vi "GLIMPSE Save image.vi"(5 "Go? (F)":bool, 7 "Header data":T1 {"Pixel depth" items=["8 bits", "16 bits", "Float", "Complex", "RGB", "HSL"]; "time of 1st frame, \nsec since 1/1/04" format="%.2f"}, 8 "Comment (for IMG file)":string, 9 "Acqisition files refnums":refnum<file>[](array[refnum]), 10 "Frame number":u32) -> (3 "Saved Image":T5)   [LabVIEW 2011]
uses:
  <vilib>/vision/Image Controls.llb/IMAQ Image.ctl
  Header file data.ctl
  Seq file v 1/Offset table.ctl
  Seq file v 1/Offset.ctl
  Seq file v 1/file number.ctl
  GLIMPSE Globals.vi
  <vilib>/vision/NI_Vision_Development_Module.lvlib
panel:
  out "Global Rectangle":i32[](array[numeric])
  in  "file path":path
  in  "File format":enum16{"TIFF", "IMG"}(ring)
  in  "stop":bool
  # "Designate an AOI to save, then press GO.\nIf no AOI is selected, the whole image will be saved."
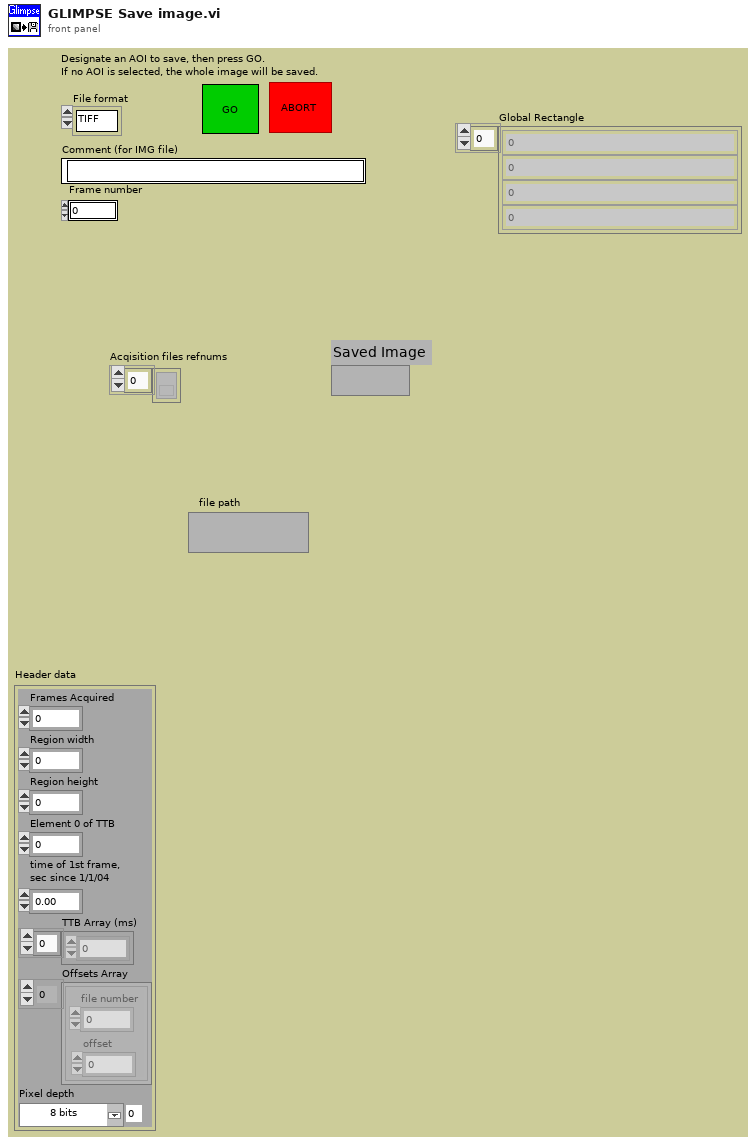
[diagram p1: front panel]
types:
  T1 = typedef "Header file data.ctl" = cluster{"Frames Acquired":u32, "Region width":i32, "Region height":i32, "Element 0 of TTB":u32, "time of 1st frame, \nsec since 1/1/04":dbl, "TTB Array (ms)":u32[], "Offsets Array":T2, "Pixel depth":u32}
  T2 = typedef "Offset table.ctl" = cluster{"offset":T3, "file number":T4}[]
  T3 = typedef "Offset.ctl" = i32
  T4 = typedef "file number.ctl" = u8
  T5 = typedef "IMAQ Image.ctl" = refnum<image>
  T6 = enum32{"No Selection", "Point", "Line", "Rectangle", "Oval", "Polygon", "Free", "Unused1", "Zoom", "Unused2", "Broken Line", "Free Hand Line"}
  T7 = enum16{"open", "open or create", "create or replace", "create"}
  T8 = enum32{"No Selection", "Point", "Line", "Rectangle", "Oval", "Polygon", "Free", "Unused1", "Zoom", "Unused2", "Broken Line", "Free Hand Line"}[]
  T9 = typedef "ROI Descriptor" = cluster{"Global Rectangle":i32[], "Contours":cluster{"ID":enum32{"External", "Internal"}, "Type":u32, "Coordinates":i32[]}[]}
  T10 = cluster{i32, i32, "X Resolution":i32, "Y Resolution":i32, dbl}
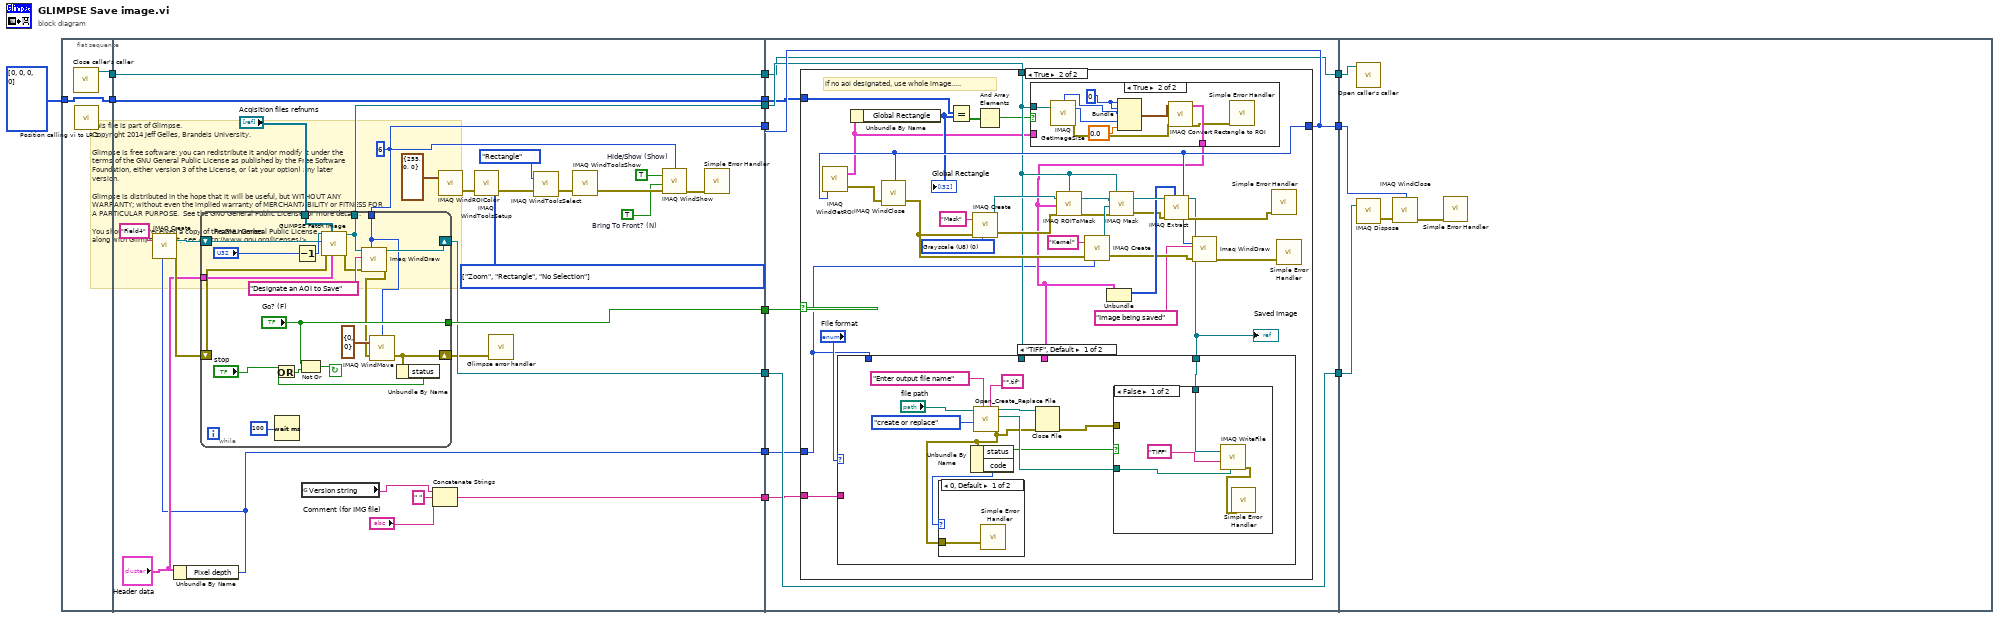
[diagram p0: block diagram]
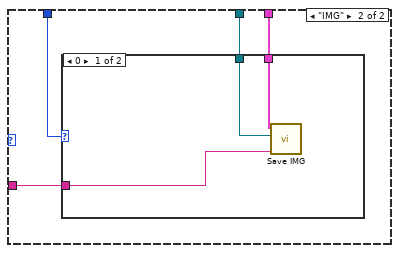
[diagram p6: hidden frame]
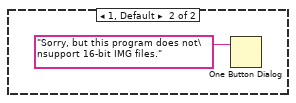
[diagram p7: hidden frame]
diagram:
  # "This file is part of Glimpse. \nCopyright 2014 Jeff Gelles, Brandeis University.    \n\nGlimpse is free software: you can redistribute it and/or modify it under the \nterms of the GNU General Public License as published by the Free Software \nFoundation, either version 3 of the License, or (at your option) any later \nversion.\n\nGlimpse is distributed in the hope that it will be useful, but WITHOUT ANY \nWARRANTY; without even the implied warranty of MERCHANTABILITY or FITNESS FOR \nA PARTICULAR PURPOSE.  See the GNU General Public License for more details.\n\nYou should have received a copy of the GNU General Public License\nalong with Glimpse.  If not, see <http://www.gnu.org/licenses/>."
  n1 = flat-sequence {
    tunnel: i32[] [0, 0, 0, 0] -> [w15]
    tunnel: [w15] -> w13
    tunnel: [w16] -> w12
    tunnel: w13 -> [w24]
    tunnel: [w24] -> w11
    tunnel: [w33] -> w10
    tunnel: [w31] -> w9
    tunnel: [w32] -> w8
    tunnel: [w28] -> w7
    tunnel: w12 -> [w23]
    tunnel: [w23] -> w6
    tunnel: [w19] -> w2
    tunnel: [w17] -> w1
    tunnel: w11 -> [w68]
    tunnel: w10 -> [w70]
    tunnel: w9 -> [w69]
    tunnel: w8 -> [w71]
    tunnel: [w71] -> w5
    tunnel: w7 -> [w67]
    tunnel: [w67] -> w4
    tunnel: w6 -> [w66]
    tunnel: [w66] -> w3
    tunnel: w2 -> [w65]
    tunnel: w1 -> [w64]
    tunnel: w5 -> [w138]
    tunnel: w4 -> [w136]
    tunnel: w3 -> [w135]
    frame #0 {
      n2 = call "Close caller's caller.vi"() -> ("vi reference"=w16:refnum<vi>)  [unwired: 1 in, 7 out]
      n3 = call "Position calling vi to LR 2.vi"() -> ()  [unwired: 2 in, 4 out]
    }
    frame #1 {
      w32 = 6 ("Window Number (0...15)")
      w35 = TRUE  # Bring To Front? (N)
      w36 = TRUE  # Hide/Show (Show)
      w41 = T8 [enum."Zoom", enum."Rectangle", enum."No Selection"] items=["No Selection", "Point", "Line", "Rectangle", "Oval", "Polygon", "Free", "Unused1", "Zoom", "Unused2", "Broken Line", "Free Hand Line"] ("Tools")
      n4 = Unbundle By Name("Header data") -> ("Pixel depth"=w17:u32)
      n5 = call "IMAQ Create"("Image Name"="Field4", "Image Type"=w17) -> ("New Image"=w29:T5, "error out"=w25:errorcluster)  [unwired: 2 in, 1 out]
      n6 = while {
        shift-left: w29 -> [w57]
        shift-right: [w55] -> w28
        tunnel: ["Go? (F)"] -> w31
        tunnel: w32 -> [w50]
        tunnel: [w58] -> w33
        tunnel: "Acqisition files refnums" -> [w53]
        shift-right: [w45] -> w26
        shift-left: w25 -> [w46]
        tunnel: "Header data" -> [w44]
        stop <- w62 continue-if-true
        n7 = Wait (ms)(milliseconds to wait=u32 100) -> ()  [unwired: 1 out]
        n8 = Decrement(x="Frame number") -> (x-1=w61:u32)
        n9 = call "GLIMPSE Fetch Image.vi"("Header file data"=w44, "Acqisition files refnums"=w53, "error in"=w46, "Logical Frame Number\n(starting with zero)"=w61, "Image In"=w57) -> ("error out"=w54:errorcluster, "Image Out"=w58:T5)  [unwired: 2 in, 3 out]
        n10 = call "Imaq WindDraw"("Window Number (0...15)"=w50, "error in (no error)"=w54, "Title"="Designate an AOI to Save", "Image"=w58) -> ("error out"=w51:errorcluster, "Image Out (duplicate)"=w55:T5)  [unwired: 2 in, 4 out]
        n11 = call "IMAQ WindMove"("Window Number (0...15)"=w50, "Coordinates (screen)"=cluster{"X Position":i32, "Y Position":i32} {"X Position"=0, "Y Position"=0}, "error in (no error)"=w51) -> ("error out"=w45:errorcluster)  [unwired: 1 in, 2 out]
        n12 = Unbundle By Name(w45) -> ("status"=w47:bool)
        n13 = Or(x="stop", y=w47) -> (x .or. y?=w49:bool)
        n14 = Not Or(1:w49, 2:"Go? (F)") -> (0:w62:bool)
      }
      n15 = global read "GLIMPSE Globals.vi" "Version string"() -> (w21:string)
      n16 = Concatenate Strings(w21, " " ("string"), "Comment (for IMG file)") -> (w19:string)
      n17 = call "IMAQ WindROIColor"("Color of ROI (white)"=cluster{"Red":u8, "Green":u8, "Blue":u8} {"Red"=255, "Green"=0, "Blue"=0}) -> ("error out"=w42:errorcluster)  [unwired: 1 in, 4 out]
      n18 = call "IMAQ WindToolsSetup"("Tools"=w41, "error in (no error)"=w42) -> ("error out"=w40:errorcluster)  [unwired: 2 in, 2 out]
      n19 = call "Glimpse error handler.vi"("error in"=w26) -> ()  [unwired: 1 in, 6 out]
      n20 = call "IMAQ WindToolsSelect"("Tool (Point)"=T6."Rectangle", "error in (no error)"=w40) -> ("error out"=w39:errorcluster)  [unwired: 2 in, 2 out]
      n21 = call "IMAQ WindToolsShow"("error in (no error)"=w39) -> ("error out"=w38:errorcluster)  [unwired: 2 in, 3 out]
      n22 = call "IMAQ WindShow"("error in (no error)"=w38, "Bring To Front? (N)"=w35, "Hide/Show (Show)"=w36, "Window Number (0...15)"=w32) -> ("error out"=w37:errorcluster)  [unwired: 1 in, 3 out]
      n23 = call <vilib>:"Simple Error Handler.vi"("error in (no error)"=w37) -> ()  [unwired: 1 in, 8 out]
    }
    frame #2 {
      n24 = case shown="True" w69 {
        tunnel: w71 -> [_ w87]
        tunnel: w70 -> [_ w79]
        tunnel: w68 -> [_ w76]
        tunnel: w65 -> [_ w74]
        tunnel: w64 -> [_ w73]
        frame False {
        }
        frame True {
          w72 = u32 0 items=["Grayscale (U8)", "Grayscale (I16)", "Grayscale (SGL)", "Complex (CSG)", "RGB (U32)", "HSL (U32)", "RGB (U64)"] ("Image Type")
          # "if no aoi designated, use whole image....."
          n25 = call "IMAQ WindGetROI"("Window Number (0...15)"=w87) -> ("ROI Descriptor"=w77:T9, "error out"=w100:errorcluster)  [unwired: 1 in, 3 out]
          n26 = Unbundle By Name(w77) -> ("Global Rectangle"=w81:i32[])
          "Global Rectangle" <- w81
          n27 = call "IMAQ WindClose"("Window Number (0...15)"=w87, "error in (no error)"=w100) -> ("error out"=w86:errorcluster)  [unwired: 1 in, 3 out]
          n28 = Equal?(x=w76, y=w81) -> (x = y?=w80:bool[])
          n29 = call "IMAQ Create"("Image Name"="Mask", "Image Type"=w72, "error in (no error)"=w86) -> ("New Image"=w98:T5, "error out"=w92:errorcluster)  [unwired: 1 in, 1 out]
          n30 = And Array Elements(Boolean array=w80) -> (logical AND=w75:bool)
          n31 = case shown="True" w75 {
            tunnel: w79 -> [_ w110]
            tunnel: [w101 w107] -> w78
            tunnel: w77 -> [w101 _]
            frame False {
            }
            frame True {
              w108 = 0
              n32 = call "IMAQ GetImageSize"("Image"=w110) -> ("Y Resolution"=w105:i32, "X Resolution"=w104:i32, "error out"=w102:errorcluster)  [unwired: 1 in, 2 out]
              n33 = Bundle(w108, w108, "X Resolution"=w104, "Y Resolution"=w105, 0.0) -> (w103:T10)  [unwired: 1 out]
              n34 = call "IMAQ Convert Rectangle to ROI"("error in (no error)"=w102, "Rectangle"=w103) -> ("error out"=w106:errorcluster, "ROI Descriptor"=w107:T9)  [unwired: 7 out]
              n35 = call <vilib>:"Simple Error Handler.vi"("error in (no error)"=w106) -> ()  [unwired: 1 in, 8 out]
            }
          }
          n36 = call "IMAQ ROIToMask"("error in (no error)"=w92, "ROI Descriptor"=w78, "Image"=w98, "Image Model"=w79) -> ("error out"=w91:errorcluster, "Image Out"=w97:T5)  [unwired: 1 in, 2 out]
          n37 = call "IMAQ Create"("Image Name"="Kernel", "Image Type"=w73, "error in (no error)"=w86) -> ("New Image"=w95:T5, "error out"=w88:errorcluster)  [unwired: 1 in, 1 out]
          n38 = Unbundle(w78) -> ("Global Rectangle"=w93:i32[])  [unwired: 1 out]
          n39 = call "IMAQ Mask"("error in (no error)"=w91, "Image Dst"=w95, "Image Mask"=w97, "Image Src"=w79) -> ("error out"=w90:errorcluster, "Image Dst Out"=w94:T5)  [unwired: 1 out]
          n40 = call "IMAQ Extract"("Optional Rectangle"=w93, "error in (no error)"=w90, "Image Src"=w94) -> ("error out"=w89:errorcluster, "Image Dst Out"=w82:T5)  [unwired: 3 in, 4 out]
          "Saved Image" <- w82
          n41 = case shown="\"TIFF\", Default" "File format" {
            tunnel: w78 -> [_ w130]
            tunnel: w79 -> [_ w129]
            tunnel: w82 -> [w121 _]
            tunnel: w73 -> [_ w128]
            tunnel: w74 -> [_ w127]
            frame "TIFF", Default {
              n42 = call <vilib>:"Open_Create_Replace File.vi"("pattern"="*.tif", "prompt"="Enter output file name", "function (open:0)"=T7."create or replace", "file path"="file path") -> ("error out"=w113:errorcluster, "new file path"=w114:path, "refnum"=w115:refnum<file>)  [unwired: 3 in, 2 out]
              n43 = Unbundle By Name(w113) -> ("status"=w112:bool, "code"=w120:i32)
              n44 = case shown="0, Default" w120 {
                tunnel: w113 -> [w126 _]
                frame 0, Default {
                  n45 = call <vilib>:"Simple Error Handler.vi"("error in (no error)"=w126) -> ()  [unwired: 1 in, 8 out]
                }
                frame 43 {
                }
              }
              n46 = Close File(refnum=w115, error in=w113) -> (error out=w111:errorcluster)  [unwired: 1 out]
              n47 = case shown="False" w112 {
                tunnel: w121 -> [w125 _]
                tunnel: w114 -> [w123 _]
                tunnel: w111 -> [_ _]
                frame False {
                  n48 = call "IMAQ WriteFile"("File Type"="TIFF", "File Path"=w123, "Image"=w125) -> ("error out"=w122:errorcluster)  [unwired: 2 in, 3 out]
                  n49 = call <vilib>:"Simple Error Handler.vi"("error in (no error)"=w122) -> ()  [unwired: 1 in, 8 out]
                }
                frame True {
                }
              }
            }
            frame "IMG" {
              n50 = case shown="0" w128 {
                tunnel: w130 -> [w133 _]
                tunnel: w129 -> [w132 _]
                tunnel: w127 -> [w131 _]
                frame 0 {
                  n51 = call "Save IMG.vi"("Comment"=w131, "Image"=w132, "ROI Descriptor"=w133) -> ()  [unwired: 2 in, 3 out]
                }
                frame 1, Default {
                  n52 = One Button Dialog(message="Sorry, but this program does not\nsupport 16-bit IMG files.") -> ()  [unwired: 2 out]
                }
              }
            }
          }
          n53 = call "Imaq WindDraw"("Window Number (0...15)"=w87, "error in (no error)"=w88, "Title"="Image being saved", "Image"=w82) -> ("error out"=w85:errorcluster)  [unwired: 2 in, 5 out]
          n54 = call <vilib>:"Simple Error Handler.vi"("error in (no error)"=w89) -> ()  [unwired: 1 in, 8 out]
          n55 = call <vilib>:"Simple Error Handler.vi"("error in (no error)"=w85) -> ()  [unwired: 1 in, 8 out]
        }
      }
    }
    frame #3 {
      n56 = call "Open caller's caller.vi"("vi reference"=w135) -> ()  [unwired: 1 in, 7 out]
      n57 = call "IMAQ Dispose"("Image"=w136) -> ("error out"=w137:errorcluster)  [unwired: 2 in, 3 out]
      n58 = call "IMAQ WindClose"("Window Number (0...15)"=w138, "error in (no error)"=w137) -> ("error out"=w139:errorcluster)  [unwired: 1 in, 3 out]
      n59 = call <vilib>:"Simple Error Handler.vi"("error in (no error)"=w139) -> ()  [unwired: 1 in, 8 out]
    }
  }
